vi "setTemperature.vi"(8 "error in (no error)":errorcluster, 10 "Period":T1, 11 "ElectrometerController in":refnum<class "ElectrometerController.lvclass">) -> (0 "error out":errorcluster, 3 "ElectrometerController out":refnum<class "ElectrometerController.lvclass">)   [LabVIEW 2016, in "ElectrometerController.lvclass"]
uses:
  ElectrometerController.lvclass
  ts_electrometeruserevents/Typedefs/MeasuringPeriod.ctl
  ElectrometerController.lvclass/ElectrometerController.ctl
  Electrometer/Electrometer.lvclass
  ts_electrometeruserevents/Typedefs/ElectrometerTypedefs.lvlib
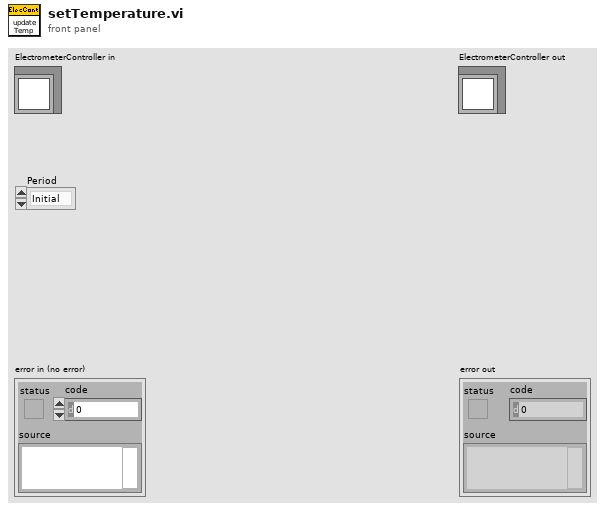
[diagram p1: front panel]
types:
  T1 = typedef "ElectrometerTypedefs.lvlib/MeasuringPeriod.ctl" = enum16{"Initial", "End"}
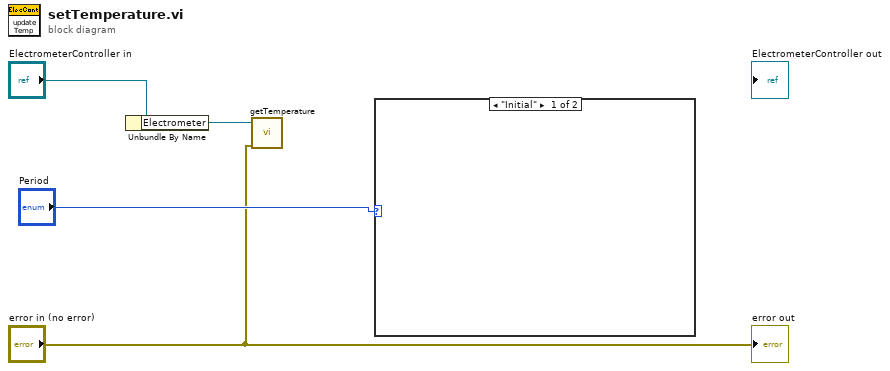
[diagram p0: block diagram]
diagram:
  n1 = Unbundle By Name("ElectrometerController in") -> ("Electrometer"=w2:refnum<class "Electrometer.lvclass">)
  n2 = call "getTemperature.vi"("error in (no error)"="error in (no error)", "Electrometer in"=w2) -> ()  [unwired: 7 in, 3 out]
  n3 = case shown="\"Initial\"" "Period" {
    frame "Initial" {
    }
    frame "End" {
    }
  }
  "error out" <- "error in (no error)"
